vi "centralizes.vi"(3 "Y in":ext[](array[numeric]), 5 "X in":ext[](array[numeric])) -> (0 "Y out":ext[](array[numeric]), 2 "X out":ext[](array[numeric]))   [LabVIEW 2014]
doc: "André Romero - 2016\nandretec@ifsc.usp.br\n\nCentralizes coordenates"
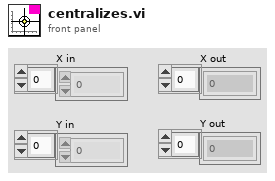
[diagram p1: front panel]
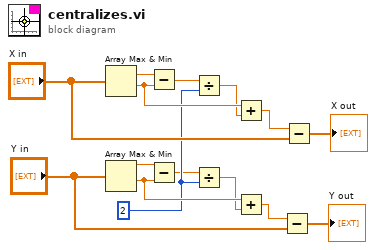
[diagram p0: block diagram]
diagram:
  w7 = 2
  n1 = Array Max & Min(array="X in") -> (max value=w3:ext, min value=w10:ext)  [unwired: 2 out]
  n2 = Array Max & Min(array="Y in") -> (max value=w4:ext, min value=w11:ext)  [unwired: 2 out]
  n3 = Subtract(x=w3, y=w10) -> (x-y=w5:ext)
  n4 = Subtract(x=w4, y=w11) -> (x-y=w6:ext)
  n5 = Divide(x=w5, y=w7) -> (x/y=w8:ext)
  n6 = Divide(x=w6, y=w7) -> (x/y=w9:ext)
  n7 = Add(x=w10, y=w8) -> (x+y=w12:ext)
  n8 = Add(x=w11, y=w9) -> (x+y=w14:ext)
  n9 = Subtract(x=w14, y="Y in") -> (x-y=→"Y out":ext[])
  n10 = Subtract(x=w12, y="X in") -> (x-y=→"X out":ext[])
